vi "ResizeArrayToPane.vi"(5 "Borders in Percent(T) or Pixels (F)":bool, 6 "Adjust":u16(ring) items=["Height", "Width", "Both"], 7 "Minimal":T1, 8 "error in (no error)":errorcluster, 9 "Borders":T2, 10 "Array":refnum<vi>, 11 "PentaPanesGUI in":refnum<class "PentaPanes.lvclass">) -> (0 "error out":errorcluster, 3 "PentaPanesGUI out":refnum<class "PentaPanes.lvclass">)   [LabVIEW 2022 SP3, in "PentaPanesLibrary.lvlib" / "PentaPanes.lvclass"]
uses:
  PentaPanes.lvclass
  BordersCluster.ctl
  <vilib>/Utility/miscctls.llb/LVBoundsTypeDef.ctl
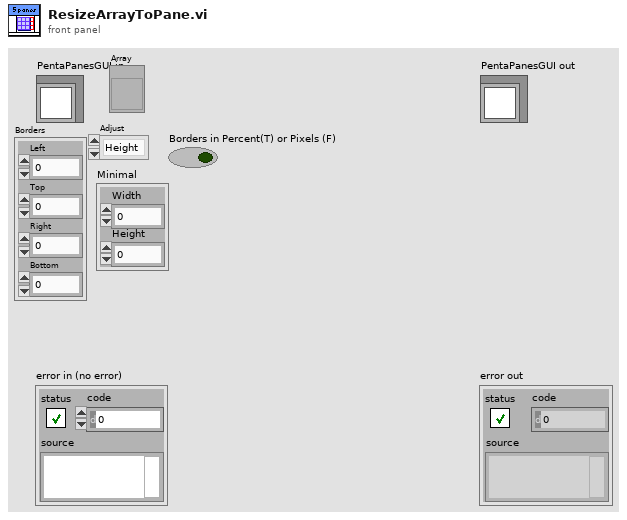
[diagram p1: front panel]
types:
  T1 = typedef "LVBoundsTypeDef.ctl" = cluster{"Width":i32, "Height":i32}
  T2 = typedef "PentaPanesLibrary.lvlib/PentaPanes.lvclass/BordersCluster.ctl" = cluster{"Left":i32, "Top":i32, "Right":i32, "Bottom":i32}
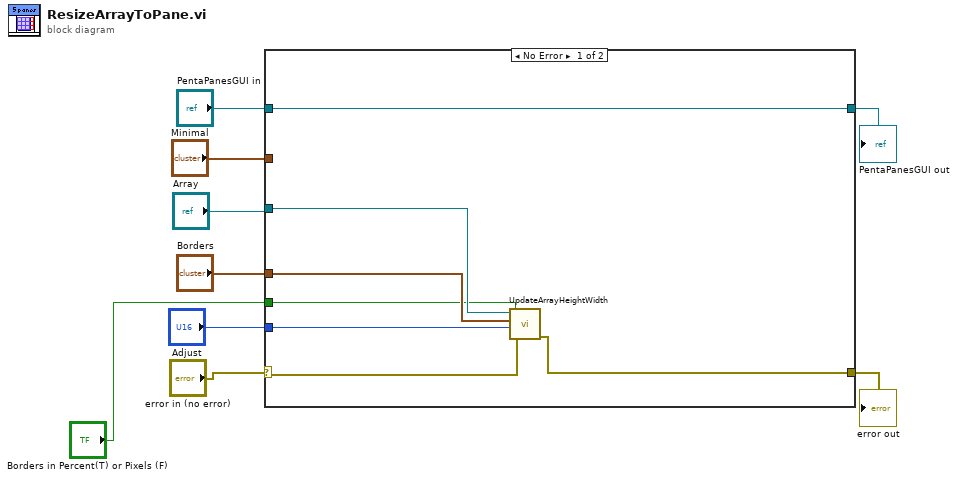
[diagram p0: block diagram]
diagram:
  n1 = case shown="No Error" "error in (no error)" {
    selector: "error in (no error)" -> [w14 w18]
    tunnel: [w13 w18] -> w8
    tunnel: [w16 w17] -> w6
    tunnel: "PentaPanesGUI in" -> [w16 w17]
    tunnel: "Array" -> [w15 _]
    tunnel: "Borders" -> [w12 _]
    tunnel: "Adjust" -> [w11 _]
    tunnel: "Minimal" -> [_ _]
    tunnel: "Borders in Percent(T) or Pixels (F)" -> [w10 _]
    frame No Error {
      n2 = call "UpdateArrayHeightWidth.vi"("Borders in Percent(T) or Pixels (F)"=w10, "error in (no error)"=w14, "Adjust"=w11, "Borders"=w12, "Array in"=w15) -> ("error out"=w13:errorcluster)  [unwired: 6 in]
    }
    frame Error {
    }
  }
  "error out" <- w8
  "PentaPanesGUI out" <- w6
